vi "Check if Data Changed.vi"(9 "Buffer":dbl[](array[numeric]), 11 "VS Data":dbl[](array[numeric])) -> (2 "Data Changed?":bool)   [LabVIEW 2021]
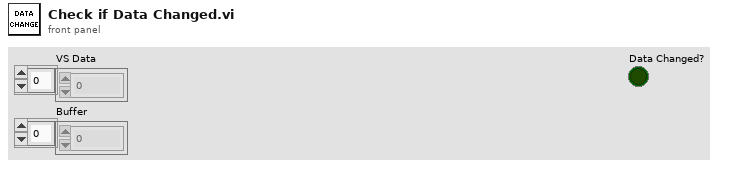
[diagram p1: front panel]
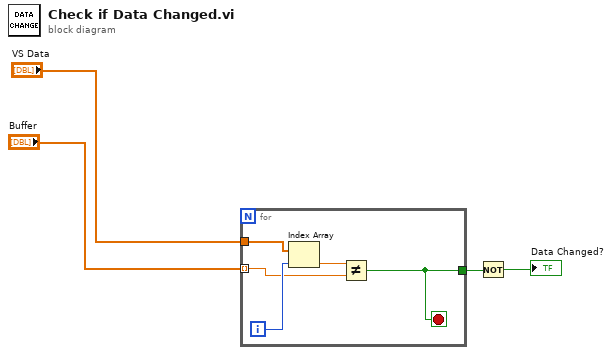
[diagram p0: block diagram]
diagram:
  n1 = for {
    tunnel: "Buffer" -> [w6] mode=indexing
    tunnel: "VS Data" -> [w9]
    tunnel: [w5] -> w2
    i -> [w8]
    stop <- w5 stop-if-true
    n2 = Index Array(array=w9, index=w8) -> (element=w7:dbl)
    n3 = Not Equal?(x=w7, y=w6) -> (x != y?=w5:bool)
  }
  n4 = Not(x=w2) -> (.not. x?=→"Data Changed?":bool)
